vi "PH_TKTDS-30xx.Evt Call Set Acquisition Configuration.vi"(0 "i ref in":refnum<vi>, 1 "Instance":string="N/A", 2 "Acquisition Configuration":T1={"Time base"=2e-07, "Record Length"=10000, "Start Time"=0.0, "Type"=1, "Continuous"=TRUE} {"Start Time" format="%#_12p"; "Record Length" items=["500"=500, "10000"=10000]; "Time base" items=["2ns"=2e-09, "4ns"=4e-09, "10ns"=1e-08, "20ns"=2e-08, "40ns"=4e-08, "100ns"=1e-07, "200ns"=2e-07, "400ns"=4e-07, "1µs"=1e-06, "2µs"=2e-06, "4µs"=4e-06, "10µs"=1e-05, "20µs"=2e-05, "40µs"=4e-05, "100µs"=0.0001, "200µs"=0.0002, "400µs"=0.0004, "1ms"=0.001, "2ms"=0.002, "10ms"=0.01, "20ms"=0.02, "40ms"=0.04, "100ms"=0.1, "200ms"=0.2, "400ms"=0.4, "1s"=1.0, "2s"=2.0, "4s"=4.0, "10s"=10.0]}, 5 "error in (no error)":errorcluster) -> (14 "i ref out":refnum<vi>, 19 "error out":errorcluster)   [LabVIEW 2014, in "PH_TKTDS-30xx.lvlib"]
doc: "This VI calls sets a simple call."
uses:
  PH_TKTDS-30xx.lvlib
  PH_TKTDS-30xx.Acquisition Config.ctl
  CS_Core/CSSystem/CoreLib/CoreLib.short 2 byte array.vi
  CS_Core/CSSystem/CoreLib/CoreLib.int 2 byte array.vi
  CS_Core/CSSystem/CoreLib/CoreLib.double 2 byte array.vi
  CS_Core/CSSystem/CoreLib/CoreLib.lvlib
  CS_Core/BaseProcess/BaseProcess.lvlib
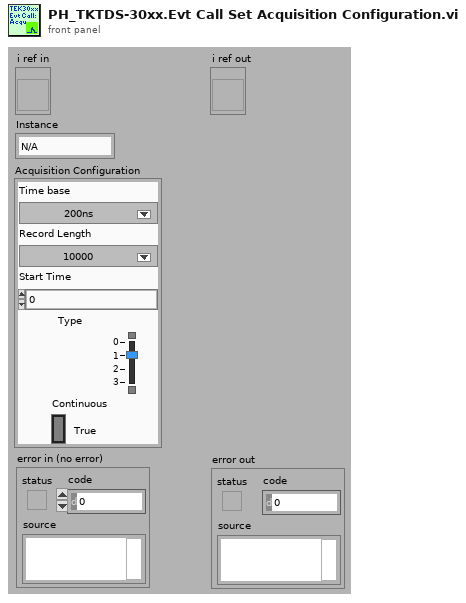
[diagram p1: front panel]
types:
  T1 = typedef "PH_TKTDS-30xx.lvlib/PH_TKTDS-30xx.Acquisition Config.ctl" = cluster{"Time base":dbl, "Record Length":u16, "Start Time":dbl, "Type":i32, "Continuous":bool}
  T2 = typedef "CoreDefs.rawDataType.ctl" = i8[]
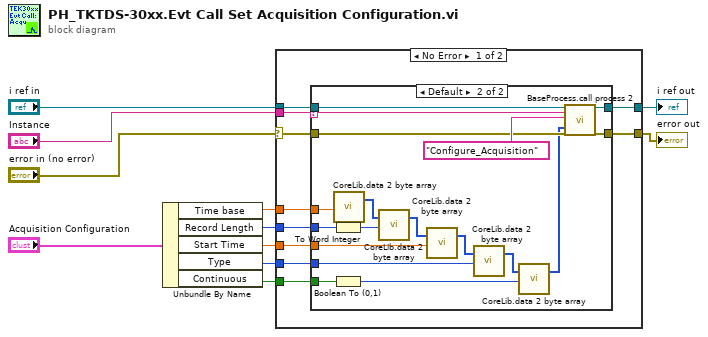
[diagram p0: block diagram]
diagram:
  n1 = Unbundle By Name("Acquisition Configuration") -> ("Time base"=w5:dbl, "Record Length"=w4:u16, "Start Time"=w3:dbl, "Type"=w2:i32, "Continuous"=w1:bool)
  n2 = case shown="No Error" "error in (no error)" {
    selector: "error in (no error)" -> [w17 w42]
    tunnel: [w21 w43] -> w11
    tunnel: [w20 w42] -> w10
    tunnel: "i ref in" -> [w19 w43]
    tunnel: w5 -> [w16 _]
    tunnel: "Instance" -> [w18 _]
    tunnel: w4 -> [w15 _]
    tunnel: w3 -> [w14 _]
    tunnel: w2 -> [w13 _]
    tunnel: w1 -> [w12 _]
    frame No Error {
      n3 = case shown="Default" w18 {
        selector: w18 -> [_ w36]
        tunnel: [w22 w40] -> w21
        tunnel: [w23 w39] -> w20
        tunnel: w19 -> [w22 w38]
        tunnel: w17 -> [w23 w37]
        tunnel: w16 -> [_ w35]
        tunnel: w15 -> [_ w34]
        tunnel: w14 -> [_ w32]
        tunnel: w13 -> [_ w29]
        tunnel: w12 -> [_ w28]
        frame "N/A" {
        }
        frame Default {
          n4 = To Word Integer(number=w34) -> (16bit integer=w24:i16)
          n5 = Boolean To (0,1)(Boolean=w28) -> (0, 1=w27:i16)
          n6 = call-poly "CoreLib.data 2 byte array.vi"("f64"=w35) -> ("byteArray out"=w33:T2)  [unwired: 18 in]
          n7 = call-poly "CoreLib.data 2 byte array.vi"("byteArray"=w33, "i16"=w24) -> ("byteArray out"=w31:T2)  [unwired: 17 in]
          n8 = call-poly "CoreLib.data 2 byte array.vi"("byteArray"=w31, "f64"=w32) -> ("byteArray out"=w26:T2)  [unwired: 17 in]
          n9 = call-poly "CoreLib.data 2 byte array.vi"("byteArray"=w26, "i32"=w29) -> ("byteArray out"=w30:T2)  [unwired: 17 in]
          n10 = call-poly "CoreLib.data 2 byte array.vi"("byteArray"=w30, "i16"=w27) -> ("byteArray out"=w25:T2)  [unwired: 17 in]
          n11 = call "BaseProcess.call process 2.vi"("i ref in"=w38, "Object"=w36, "Selector"="Configure_Acquisition", "Data"=w25, "error in (no error)"=w37) -> ("i ref out"=w40:refnum<vi>, "error out"=w39:errorcluster)  [unwired: 13 in]
        }
      }
    }
    frame Error {
    }
  }
  "i ref out" <- w11
  "error out" <- w10
